vi "Send_Trajectory.vi"(8 "error in (no error)":errorcluster, 9 "Advanced":bool, 10 "Trajectory":T1) -> (0 "error out":errorcluster)   [LabVIEW 2019, in "Kinova MICO² USB.lvlib"]
uses:
  <vilib>/Utility/error.llb/Error Cluster From Error Code.vi
  <vilib>/ErrorRing/Error Ring.xnode
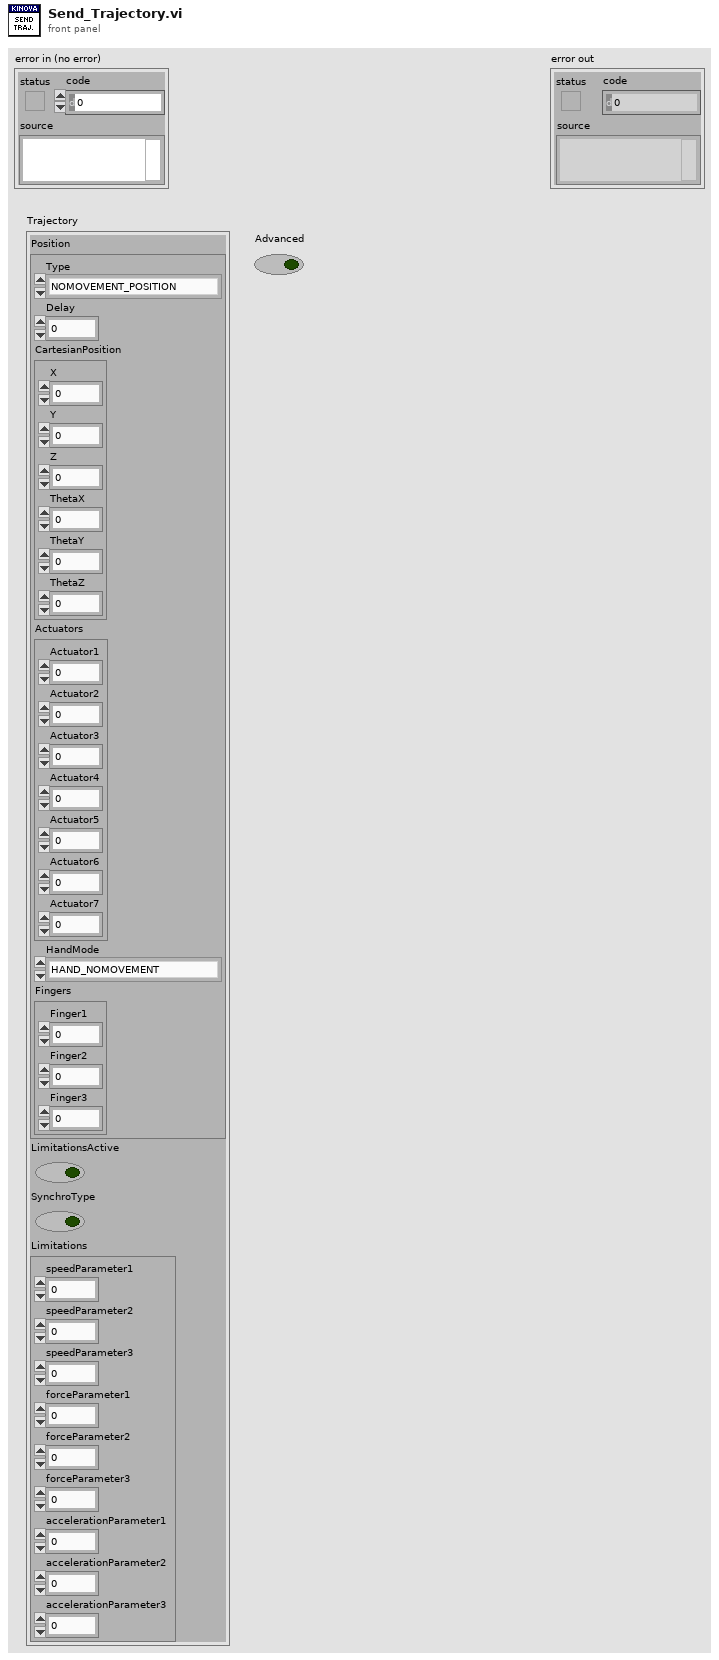
[diagram p1: front panel]
types:
  T1 = cluster{"Position":cluster{"Type":enum16{"NOMOVEMENT_POSITION", "CARTESIAN_POSITION", "ANGULAR_POSITION", "RETRACTED", "PREDEFINED1", "PREDEFINED2", "PREDEFINED3", "CARTESIAN_VELOCITY", "ANGULAR_VELOCITY", "PREDEFINED4", "PREDEFINED5", "ANY_TRAJECTORY", "TIME_DELAY"}, "Delay":sgl, "CartesianPosition":cluster{"X":sgl, "Y":sgl, "Z":sgl, "ThetaX":sgl, "ThetaY":sgl, "ThetaZ":sgl}, "Actuators":cluster{"Actuator1":sgl, "Actuator2":sgl, "Actuator3":sgl, "Actuator4":sgl, "Actuator5":sgl, "Actuator6":sgl, "Actuator7":sgl}, "HandMode":enum16{"HAND_NOMOVEMENT", "POSITION_MODE", "VELOCITY_MODE", "NO_FINGER", "ONE_FINGER", "TWO_FINGERS", "THREE_FINGERS"}, "Fingers":cluster{"Finger1":sgl, "Finger2":sgl, "Finger3":sgl}}, "LimitationsActive":bool, "SynchroType":bool, "Limitations":cluster{"speedParameter1":sgl, "speedParameter2":sgl, "speedParameter3":sgl, "forceParameter1":sgl, "forceParameter2":sgl, "forceParameter3":sgl, "accelerationParameter1":sgl, "accelerationParameter2":sgl, "accelerationParameter3":sgl}}
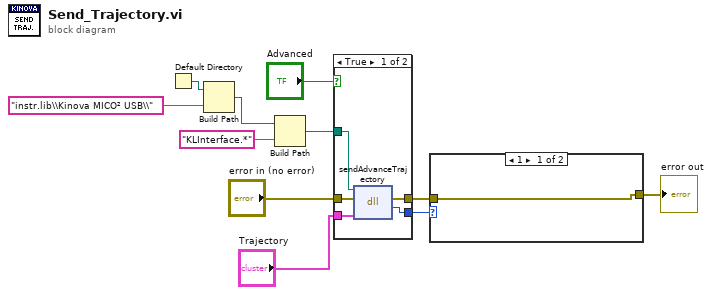
[diagram p0: block diagram]
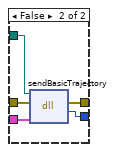
[diagram p2: hidden frame]
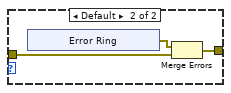
[diagram p3: hidden frame]
diagram:
  n1 = Default Directory() -> (w3:path)
  n2 = Build Path(base path=w3, name or relative path="instr.lib\\Kinova MICO² USB\\") -> (appended path=w1:path)
  n3 = Build Path(base path=w1, name or relative path="KLInterface.*") -> (appended path=w5:path)
  n4 = case shown="True" "Advanced" {
    tunnel: "error in (no error)" -> [w16 w21]
    tunnel: [w15 w20] -> w9
    tunnel: [w14 w19] -> w8
    tunnel: "Trajectory" -> [w13 w18]
    tunnel: w5 -> [w12 w17]
    frame True {
      n5 = dll-call lib="C:/Users/mcjssdcc/source/repos/Kinova Labview Interface/Debug/KLInterface.dll" fn="sendAdvanceTrajectory"(path in=w12, error in=w16, "point"=w13) -> (error out=w15:errorcluster, "return type"=w14:i32)  [unwired: 2 in, 1 out]
    }
    frame False {
      n6 = dll-call lib="C:/Users/mcjssdcc/source/repos/Kinova Labview Interface/Debug/KLInterface.dll" fn="sendBasicTrajectory"(path in=w17, error in=w21, "point"=w18) -> (error out=w20:errorcluster, "return type"=w19:i32)  [unwired: 2 in, 1 out]
    }
  }
  n7 = case shown="1" w8 {
    tunnel: [w22 w24] -> w7
    tunnel: w9 -> [w22 w23]
    frame 1 {
    }
    frame Default {
      n8 = xnode "Error Ring"() -> ("error out"=w25:errorcluster)
      n9 = Merge Errors(w25, w23) -> (w24:errorcluster)
    }
  }
  "error out" <- w7
